vi "Duplicate Disabled Frame.vi"(8 "Error In":errorcluster) -> (0 "Error Out":errorcluster)   [LabVIEW 2018, in "Toolkit.lvlib" / "Tests.lvlib"]
uses:
  src/Toolkit/Tests/Tests.lvlib
  <vilib>/Utility/traverseref.llb/TRef TravTarget.ctl
  <vilib>/addons/_JKI Toolkits/Caraya/classes/Test/Test.lvclass
  <vilib>/Utility/traverseref.llb/VI Scripting - Traverse.lvlib
  <vilib>/addons/_JKI Toolkits/Caraya/classes/Assert/Assert.lvclass
  src/Toolkit/Toolkit.lvlib
  Tests.lvlib
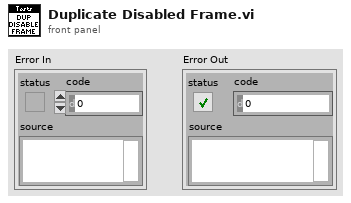
[diagram p1: front panel]
types:
  T1 = typedef "TRef TravTarget.ctl" = enum16{"FP", "BD", "Other"}
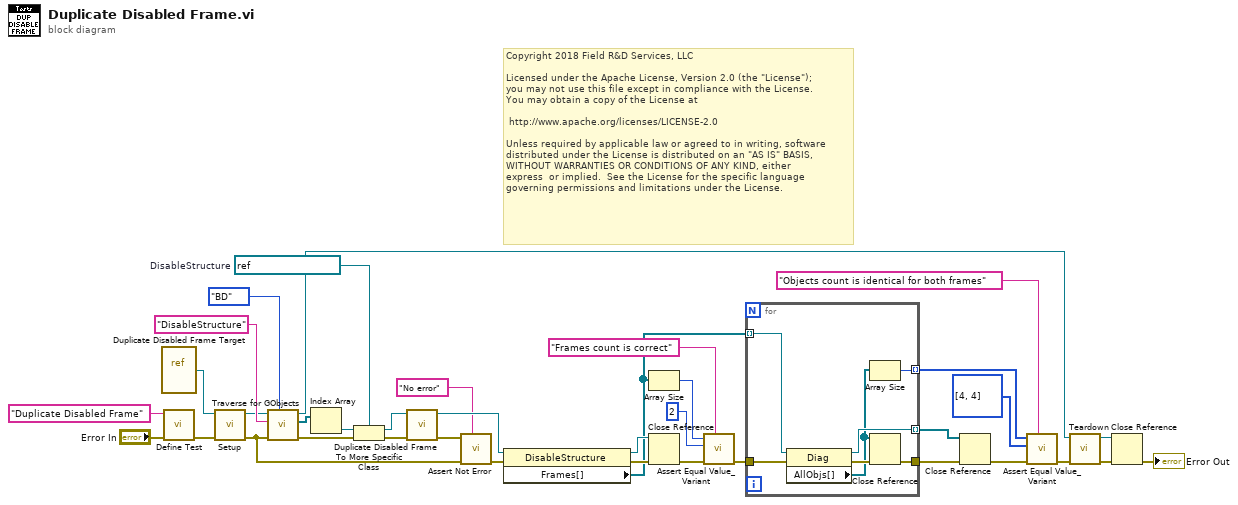
[diagram p0: block diagram]
diagram:
  w31 = refnum<vi> refnum  # DisableStructure
  # "Copyright 2018 Field R&D Services, LLC\n\nLicensed under the Apache License, Version 2.0 (the \"License\");\nyou may not use this file except in compliance with the License.\nYou may obtain a copy of the License at\n\n\thttp://www.apache.org/licenses/LICENSE-2.0\n\nUnless required by applicable law or agreed to in writing, software\ndistributed under the License is distributed on an \"AS IS\" BASIS,\nWITHOUT WARRANTIES OR CONDITIONS OF ANY KIND, either \nexpress  or implied.  See the License for the specific language \ngoverning permissions and limitations under the License."
  n1 = vi-ref "Duplicate Disabled Frame Target.vi"() -> (w29:refnum<vi>)
  n2 = call <vilib>:"Define Test.vi"("error in (no error)"="Error In", "Label (VI Title)"="Duplicate Disabled Frame") -> ("error out"=w21:errorcluster)  [unwired: 9 in]
  n3 = call "Setup.vi"("Error In"=w21, "VI In"=w29) -> ("Error Out"=w16:errorcluster, "VI Out"=w28:refnum<vi>)  [unwired: 8 in]
  n4 = call <vilib>:"Traverse for GObjects.vi"("Traverse Target"=TRef_TravTarget."BD", "error in (no error)"=w16, "Class Name"="DisableStructure", "VI Refnum"=w28) -> ("error out"=w34:errorcluster, "References"=w33:refnum<vi>[], "dup VI Refnum"=w27:refnum<vi>)  [unwired: 4 in, 1 out]
  n5 = Index Array(array=w33) -> (element=w32:refnum<vi>)  [unwired: 1 in]
  n6 = To More Specific Class(target class=w31, reference=w32, error in=w34) -> (specific class reference=w30:refnum<vi>, error out=w17:errorcluster)
  n7 = call "Duplicate Disabled Frame.vi"("Error In"=w17, "DisableStructure In"=w30) -> ("Error Out"=w13:errorcluster, "DisableStructure Out"=w23:refnum<vi>)  [unwired: 8 in]
  n8 = call <vilib>:"Assert Not Error.vi"("Label"="No error", "error in (no error)"=w16, "Not Error?"=w13) -> ("error out"=w15:errorcluster)  [unwired: 8 in]
  n9 = property class="DisableStructure"(reference=w23, error in=w15) -> (reference out=w22:refnum<vi>, error out=w20:errorcluster, "Frames[]"=w7:refnum<vi>[])
  n10 = Array Size(array=w7) -> (size(s)=w10:i32)
  n11 = Close Reference(reference=w22, error in (no error)=w20) -> (error out=w14:errorcluster)
  n12 = call <vilib>:"Assert Equal Value_Variant.vi"("Label"="Frames count is correct", "error in (no error)"=w14, "Y"=2 ("size(s)"), "X"=w10) -> ("error out"=w6:errorcluster)  [unwired: 7 in]
  n13 = for {
    tunnel: w7 -> [w44] mode=indexing
    tunnel: w6 -> [w43]
    tunnel: [w42] -> w2 mode=indexing
    tunnel: [w41] -> w4 mode=indexing
    tunnel: [w39] -> w5
    n14 = property class="Diag"(reference=w44, error in=w43) -> (reference out=w41:refnum<vi>, error out=w40:errorcluster, "AllObjs[]"=w38:refnum<vi>[])
    n15 = Array Size(array=w38) -> (size(s)=w42:i32)
    n16 = Close Reference(reference=w38, error in (no error)=w40) -> (error out=w39:errorcluster)
  }
  n17 = Close Reference(reference=w4, error in (no error)=w5) -> (error out=w3:errorcluster)
  n18 = call <vilib>:"Assert Equal Value_Variant.vi"("Label"="Objects count is identical for both frames", "error in (no error)"=w3, "Y"=i32[] [4, 4], "X"=w2) -> ("error out"=w18:errorcluster)  [unwired: 7 in]
  n19 = call "Teardown.vi"("Error In"=w18, "VI In"=w27) -> ("Error Out"=w25:errorcluster, "VI Out"=w26:refnum<vi>)  [unwired: 8 in]
  n20 = Close Reference(reference=w26, error in (no error)=w25) -> (error out=→"Error Out":errorcluster)
